vi "Retrieve_ITX_Waves.vi"() -> ()   [LabVIEW 2016]
panel:
  out "Wave Clusters":T1(array[cluster])
  out "Comments Array":string[](array[string])
  in  "length":i32=1
  in  "offset":i32
  in  "File or Folder Path":path=path "C:/"
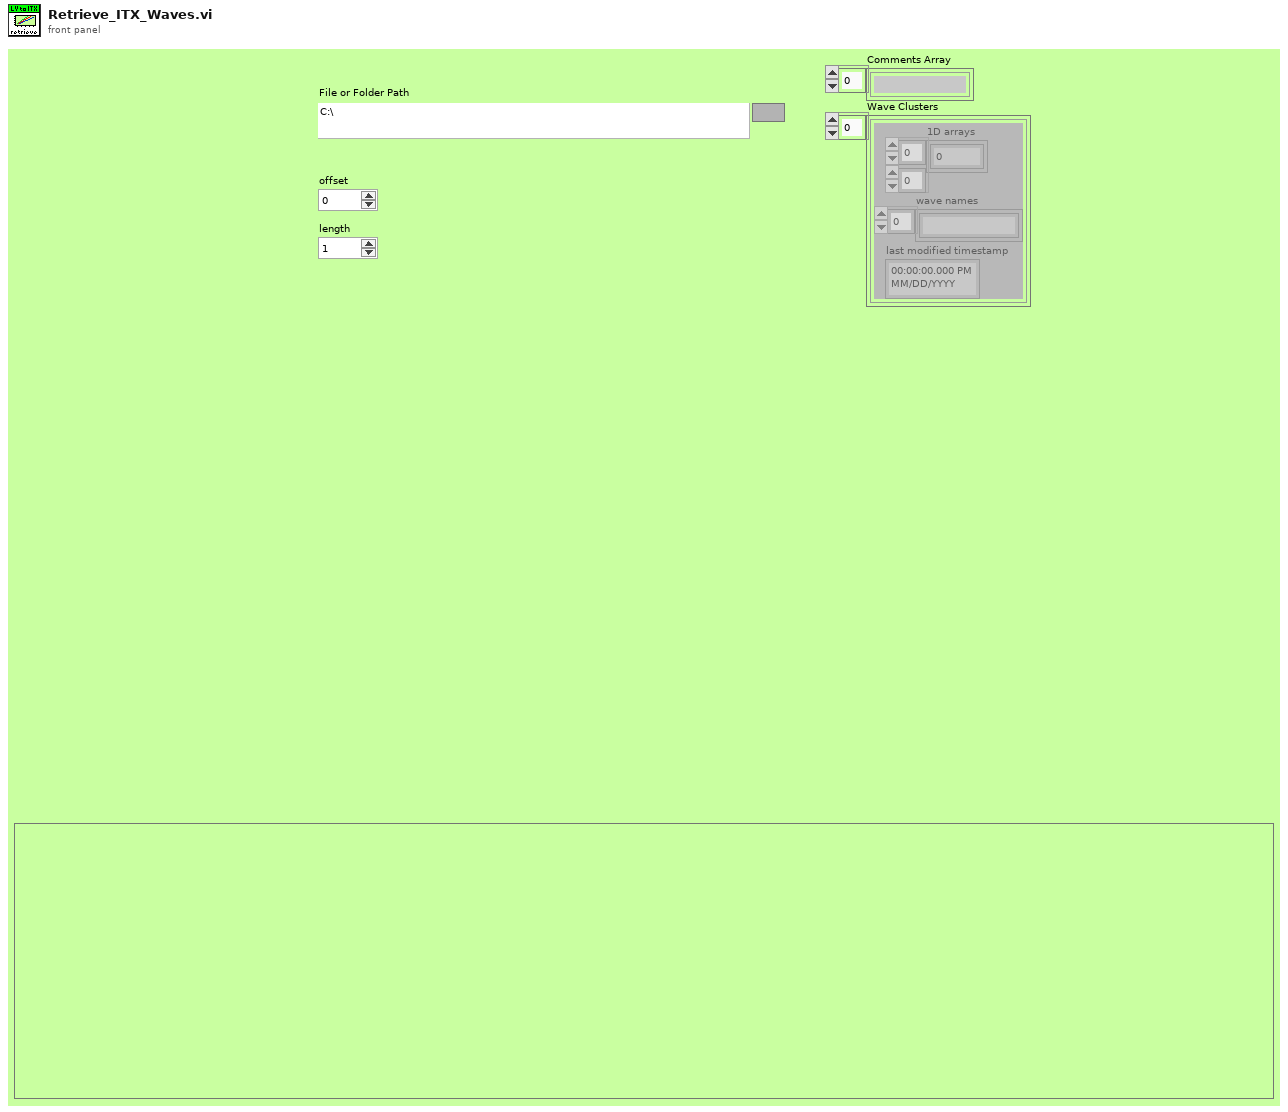
[diagram p1: front panel]
types:
  T1 = cluster{"1D arrays":dbl[][], "wave names":string[], "last modified timestamp":timestamp}[]
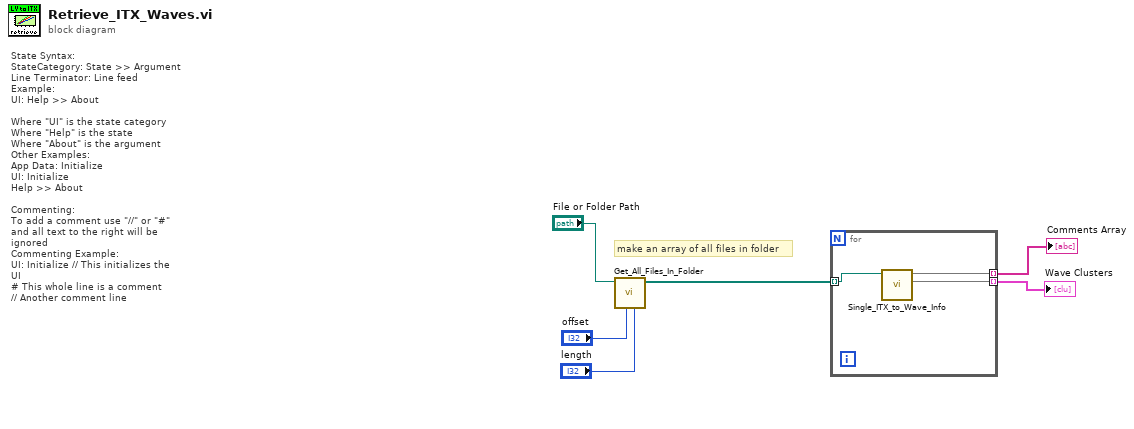
[diagram p0: block diagram]
diagram:
  # "make an array of all files in folder"
  # "State Syntax:\nStateCategory: State >> Argument\nLine Terminator: Line feed\nExample:\nUI: Help >> About\n\nWhere \"UI\" is the state category\nWhere \"Help\" is the state\nWhere \"About\" is the argument\nOther Examples:\nApp Data: Initialize\nUI: Initialize\nHelp >> About\n\nCommenting:\nTo add a comment use \"//\" or \"#\" and all text to the right will be ignored\nCommenting Example:\nUI: Initialize // This initializes the UI\n# This whole line is a comment\n// Another comment line"
  n1 = call "Get_All_Files_In_Folder.vi"("length"="length", "offset (for subset of folder)"="offset", "File or Folder Path"="File or Folder Path") -> ("array of files"=w5:path[])  [unwired: 6 in, 2 out]
  n2 = for {
    tunnel: w5 -> [w7] mode=indexing
    tunnel: [w9] -> w4 mode=indexing
    tunnel: [w8] -> w3 mode=indexing
    n3 = call "Single_ITX_to_Wave_Info.vi"("Path"=w7) -> (2:w8, 3:w9)  [unwired: 9 in]
  }
  "Comments Array" <- w4
  "Wave Clusters" <- w3
